vi "capture_dual_color_dual_view (SubVI).vi"(0 "SpimA path":path, 1 "Control values":T1, 2 "volume number":i32, 3 "filename prefix":string, 4 "Cam A handle in":u32, 5 "Capture on/off":bool, 6 "Cam A error in":errorcluster, 7 "Cam B error in":errorcluster, 8 "SpimB path":path, 10 "Cam B handle in":u32) -> (12 "Stage 0":u32, 14 "Stage 1":u32, 16 "Stage 2":u32, 18 "Stage 3":u32, 19 "Cam B Frame Count":i32, 20 "Camera A error out":errorcluster, 21 "DAC card stage A error":errorcluster, 22 "DAC card stage B error":errorcluster, 23 "interstage":u32, 24 "Camera A handle":u32, 25 "Camera B handle":u32, 26 "Cam A Frame Count":i32, 27 "Camera B error out":errorcluster)   [LabVIEW 2016]
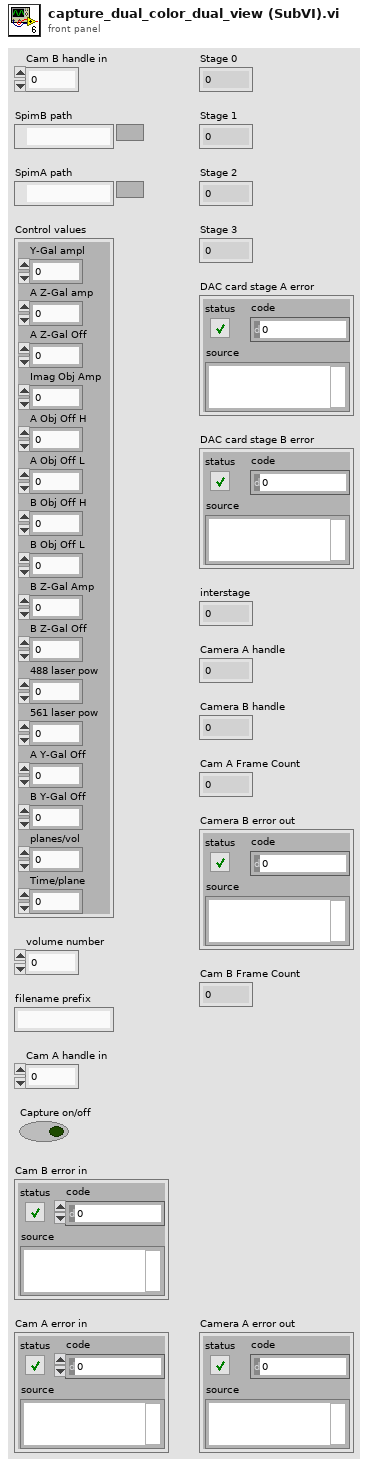
[diagram p1: front panel]
types:
  T1 = cluster{"Y-Gal ampl":dbl, "A Z-Gal amp":dbl, "A Z-Gal Off":dbl, "Imag Obj Amp":dbl, "A Obj Off H":dbl, "A Obj Off L":dbl, "B Obj Off H":dbl, "B Obj Off L":dbl, "B Z-Gal Amp":dbl, "B Z-Gal Off":dbl, "488 laser pow":dbl, "561 laser pow":dbl, "A Y-Gal Off":dbl, "B Y-Gal Off ":dbl, "planes/vol":dbl, "Time/plane":dbl}
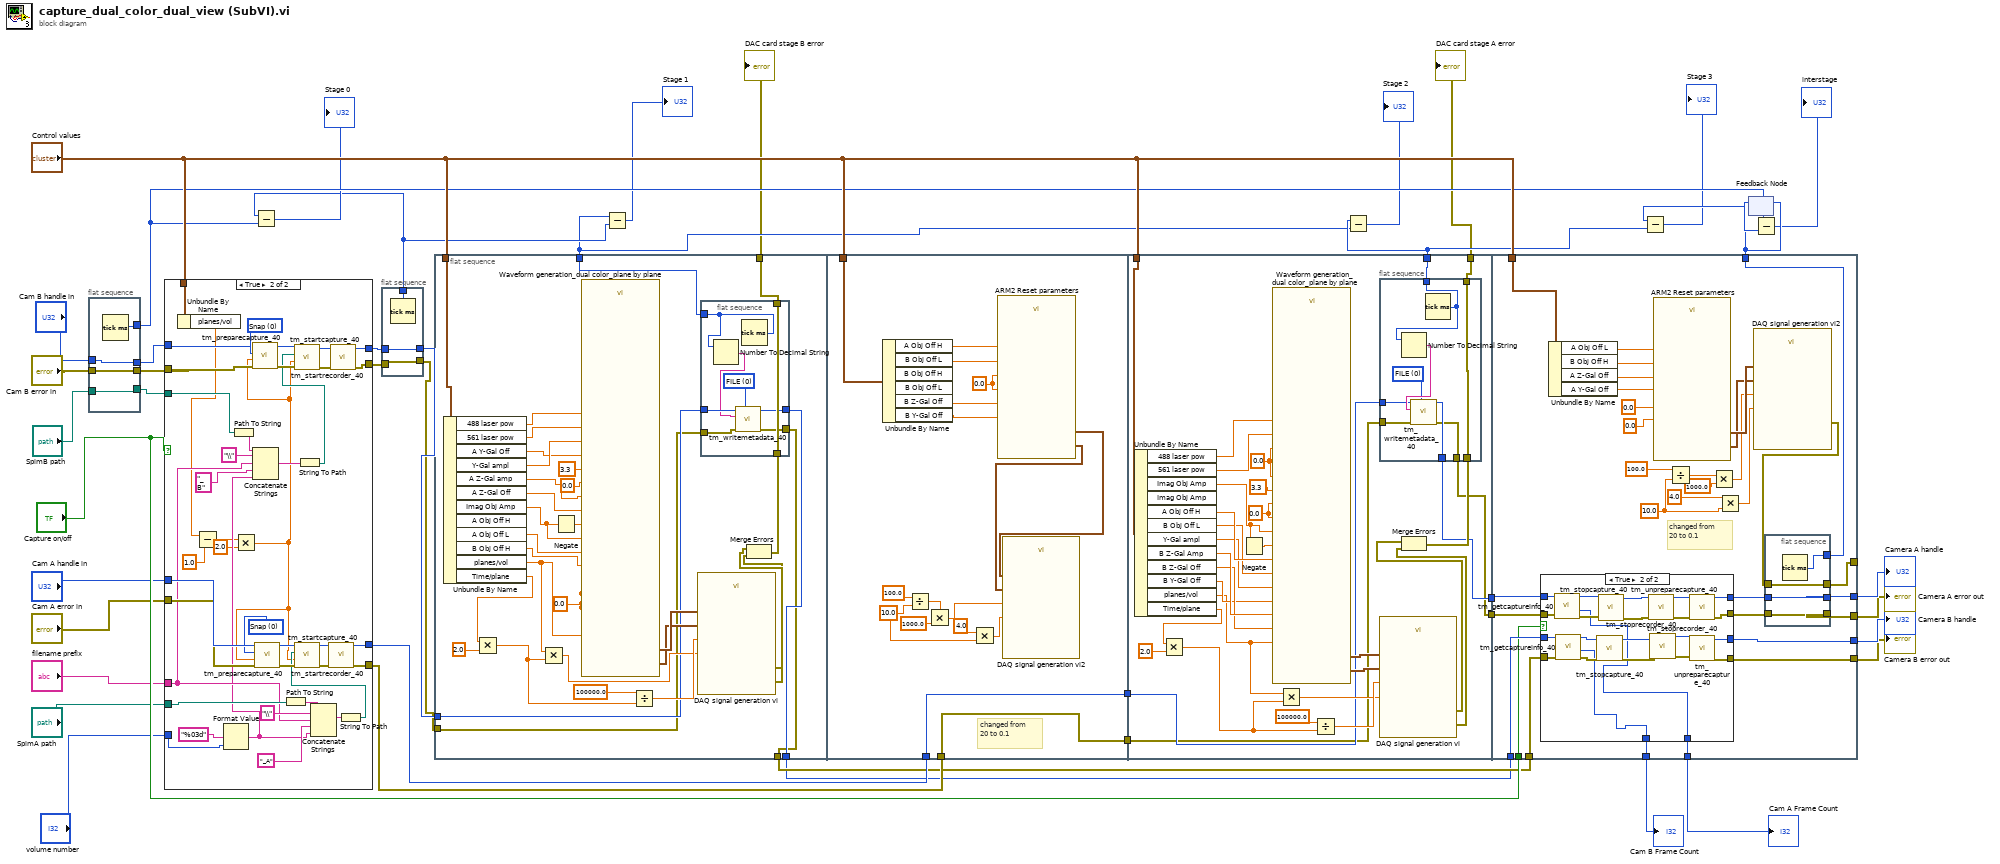
[diagram p0: block diagram]
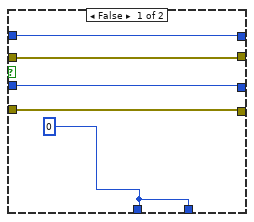
[diagram p3: hidden frame]
diagram:
  n1 = flat-sequence {
    tunnel: [w48] -> w19
    tunnel: "Cam B handle in" -> [w48]
    tunnel: [w47] -> w21
    tunnel: "Cam B error in" -> [w47]
    tunnel: [w46] -> w26
    tunnel: [w45] -> w35
    tunnel: "SpimB path" -> [w45]
    frame #0 {
      n2 = Tick Count (ms)() -> (millisecond timer value=w46:u32)
    }
  }
  n3 = case shown="True" "Capture on/off" {
    tunnel: "Cam A handle in" -> [w50 w86]
    tunnel: "Cam A error in" -> [w49 w85]
    tunnel: [w50 w77] -> w31
    tunnel: [w49 w75] -> w32
    tunnel: [w52 w82] -> w9
    tunnel: [w51 w81] -> w10
    tunnel: w19 -> [w52 w80]
    tunnel: w21 -> [w51 w79]
    tunnel: "SpimA path" -> [_ w68]
    tunnel: "volume number" -> [_ w67]
    tunnel: "filename prefix" -> [_ w60]
    tunnel: w35 -> [_ w58]
    tunnel: "Control values" -> [_ w57]
    frame False {
    }
    frame True {
      w83 = 0 items=["Snap", "Sequence"] ("Capture mode")
      w84 = 0 items=["Snap", "Sequence"] ("Capture mode")
      n4 = Unbundle By Name(w57) -> ("planes/vol"=w56:dbl)
      n5 = Subtract(x=w56, y=1.0) -> (x-y=w55:dbl)
      n6 = Format Value(format string="%03d", value (0)=w67) -> (output string=w59:string)  [unwired: 1 in]
      n7 = Path To String(path=w58) -> (string=w64:string)
      n8 = Multiply(x=w55, y=2.0) -> (x*y=w53:dbl)
      n9 = call <userlib>:"tm_preparecapture_40.vi"("error in (no error)"=w79, "Frames"=w53, "Capture mode"=w84, "Handle in"=w80) -> ("error out"=w90:errorcluster, "Handle out"=w89:u32)  [unwired: 4 in, 2 out]
      n10 = Concatenate Strings(w64, "\\", w60, "_B" ("string"), w59) -> (w63:string)
      n11 = call <userlib>:"tm_preparecapture_40.vi"("error in (no error)"=w85, "Frames"=w53, "Capture mode"=w83, "Handle in"=w86) -> ("error out"=w88:errorcluster, "Handle out"=w87:u32)  [unwired: 4 in, 2 out]
      n12 = Path To String(path=w68) -> (string=w72:string)
      n13 = String To Path(string=w63) -> (path=w61:path)
      n14 = call <userlib>:"tm_startrecorder_40.vi"("error in (no error)"=w90, "frames"=w53, "File"=w61, "Handle in"=w89) -> ("error out"=w92:errorcluster, "Handle out"=w91:u32)  [unwired: 6 in]
      n15 = Concatenate Strings(w72, "\\", w60, "_A" ("string"), w59) -> (w73:string)
      n16 = call <userlib>:"tm_startcapture_40.vi"("error in (no error)"=w92, "Handle in"=w91) -> ("error out"=w81:errorcluster, "Handle out"=w82:u32)  [unwired: 8 in]
      n17 = String To Path(string=w73) -> (path=w69:path)
      n18 = call <userlib>:"tm_startrecorder_40.vi"("error in (no error)"=w88, "frames"=w53, "File"=w69, "Handle in"=w87) -> ("error out"=w76:errorcluster, "Handle out"=w78:u32)  [unwired: 6 in]
      n19 = call <userlib>:"tm_startcapture_40.vi"("error in (no error)"=w76, "Handle in"=w78) -> ("error out"=w75:errorcluster, "Handle out"=w77:u32)  [unwired: 8 in]
    }
  }
  n20 = Subtract(x=w23, y=w26) -> (x-y=→"Stage 0":u32)
  n21 = flat-sequence {
    tunnel: [w95] -> w30
    tunnel: w9 -> [w95]
    tunnel: [w94] -> w28
    tunnel: w10 -> [w94]
    tunnel: [w93] -> w23
    frame #0 {
      n22 = Tick Count (ms)() -> (millisecond timer value=w93:u32)
    }
  }
  n23 = flat-sequence {
    tunnel: [w116] -> w3
    tunnel: [w112] -> w27
    tunnel: [w115] -> w13
    tunnel: w28 -> [w111]
    tunnel: [w110] -> w29
    tunnel: w30 -> [w113]
    tunnel: "Control values" -> [w109]
    tunnel: w31 -> [w142]
    tunnel: w32 -> [w141]
    tunnel: [w142] -> w44
    tunnel: [w141] -> w43
    tunnel: "Control values" -> [w140]
    tunnel: [w172] -> w42
    tunnel: [w171] -> w41
    tunnel: [w174] -> w8
    tunnel: [w173] -> w14
    tunnel: w44 -> [w170]
    tunnel: w43 -> [w169]
    tunnel: "Control values" -> [w167]
    tunnel: w42 -> [w223]
    tunnel: w41 -> [w222]
    tunnel: w29 -> [w224]
    tunnel: [w221] -> w4
    tunnel: [w220] -> w5
    tunnel: [w208] -> w6
    tunnel: [w206] -> w7
    tunnel: [w204] -> w17
    tunnel: [w203] -> _
    tunnel: w27 -> [w201]
    tunnel: "Control values" -> [w200]
    tunnel: "Capture on/off" -> [w195]
    tunnel: [w194] -> w39
    tunnel: [w193] -> w40
    frame #0 {
      w127 = 0.0 ("ARM2 Z-offset")
      n24 = Unbundle By Name(w109) -> ("488 laser pow"=w100:dbl, "561 laser pow"=w101:dbl, "A Y-Gal Off"=w102:dbl, "Y-Gal ampl"=w108:dbl, "A Z-Gal amp"=w107:dbl, "A Z-Gal Off"=w106:dbl, "Imag Obj Amp"=w105:dbl, "A Obj Off L"=w104:dbl, "B Obj Off H"=w103:dbl, "planes/vol"=w99:dbl, "Time/plane"=w97:dbl)  [unwired: 1 out]
      n25 = Multiply(x=w97, y=2.0) -> (x*y=w96:dbl)
      n26 = Multiply(x=w99, y=w96) -> (x*y=w121:dbl)
      n27 = Negate(x=w105) -> (-x=w114:dbl)
      n28 = call "Waveform generation_dual color_plane by plane.vi"("Number of Steps"=w99, "488 LASER Intensity"=w100, "SPIMA Obj Ampl"=w114, "SPIMB Z- galvo amplitude"=w127, "SPIMA Z-Galvo Offset"=w106, "SPIMA Z-Galvo Amplitude"=w107, "SPIMA Camera trigger"=0.0 ("ARM2 Camera trigger"), "SPIMA Obejective Offset"=w104, "SPIMB Obejective Offset"=w103, "SPIMA Y-Galvo Offset"=w102, "SPIMB Camera Trigger"=3.3 ("ARM1 Camera Trigger"), "561 Laser Amplitude"=w101, "SPIMB Objective Amplitude"=w105, "SPIMA Y-Galvo Amplitude"=w108, "SPIMB Z-offset"=w127, "SPIMB Y Offset"=w127, "SPIMB Y Amplitude"=w127) -> ("DAQ 2"=w125:waveform(dbl)[], "DAQ1"=w124:waveform(dbl)[])  [unwired: 9 in]
      n29 = Divide(x=100000.0, y=w96) -> (x/y=w122:dbl)
      n30 = call "DAQ signal generation vi.vi"("Time for each step"=w122, "Total time"=w121, "DAQ 1"=w124, "DAQ 2"=w125) -> ("error out"=w120:errorcluster, "error out 7"=w119:errorcluster)  [unwired: 6 in]
      n31 = flat-sequence {
        tunnel: w117 -> [w135]
        tunnel: [w135] -> w116
        tunnel: [w129] -> w115
        tunnel: w113 -> [w134]
        tunnel: [w133] -> w112
        tunnel: w111 -> [w132]
        tunnel: [w131] -> w110
        frame #0 {
          w130 = 0 items=["FILE"=0, "FRAME"=2] ("Type")
          n32 = Tick Count (ms)() -> (millisecond timer value=w129:u32)
          n33 = Number To Decimal String(number=w129) -> (decimal integer string=w128:string)  [unwired: 1 in]
          n34 = call <userlib>:"tm_writemetadata_40.vi"("Type"=w130, "error in (no error)"=w132, "Metadata"=w128, "Handle"=w134) -> ("error out"=w131:errorcluster, "Handle"=w133:u32)  [unwired: 6 in]
        }
      }
      n35 = Merge Errors(w120, w119) -> (w117:errorcluster)
    }
    frame #1 {
      w145 = 0.0 ("ARM1 Z-Galvo Offset")
      w149 = 10.0 ("y")
      # "changed from 20 to 0.1"
      n36 = Unbundle By Name(w140) -> ("A Obj Off H"=w139:dbl, "B Obj Off L"=w138:dbl, "B Z-Gal Off"=w137:dbl, "B Y-Gal Off"=w136:dbl)  [unwired: 2 out]
      n37 = Divide(x=100.0, y=w149) -> (x/y=w152:dbl)
      n38 = Multiply(x=w152, y=1000.0) -> (x*y=w147:dbl)
      n39 = Multiply(x=4.0, y=w149) -> (x*y=w146:dbl)
      n40 = call "ARM2 Reset parameters.vi"("ARM2 Y-Galvo Offset"=w136, "ARM2 Obejective Offset"=w138, "ARM2 Z-Galvo Offset"=w137, "ARM1 Z-Galvo Offset"=w145, "ARM1 Obejective Offset"=w139, "ARM1 Y-Galvo Offset"=w145) -> ("DAQ 2"=w144:waveform(dbl)[], "DAQ1"=w143:waveform(dbl)[])  [unwired: 8 in]
      n41 = call "DAQ signal generation vi2.vi"("Time for each step"=w147, "Total time"=w146, "DAQ1"=w143, "DAQ 2"=w144) -> ()  [unwired: 6 in, 2 out]
    }
    frame #2 {
      w168 = 0.0 ("SPIMB Camera Trigger")
      w176 = 0.0 ("ARM1 Y-Galvo Offset")
      n42 = Unbundle By Name(w167) -> ("488 laser pow"=w159:dbl, "561 laser pow"=w160:dbl, "Imag Obj Amp"=w157:dbl, "A Obj Off H"=w166:dbl, "B Obj Off L"=w165:dbl, "Y-Gal ampl"=w163:dbl, "B Z-Gal Amp"=w164:dbl, "B Z-Gal Off"=w162:dbl, "B Y-Gal Off"=w158:dbl, "planes/vol"=w156:dbl, "Time/plane"=w154:dbl)  [unwired: 1 out]
      n43 = Multiply(x=w154, y=2.0) -> (x*y=w153:dbl)
      n44 = Negate(x=w157) -> (-x=w161:dbl)
      n45 = call "Waveform generation_dual color_plane by plane.vi"("Number of Steps"=w156, "488 LASER Intensity"=w159, "SPIMA Obj Ampl"=w157, "SPIMB Z- galvo amplitude"=w164, "SPIMA Z-Galvo Offset"=w176, "SPIMA Z-Galvo Amplitude"=w176, "SPIMA Camera trigger"=3.3 ("ARM2 Camera trigger"), "SPIMA Obejective Offset"=w166, "SPIMB Obejective Offset"=w165, "SPIMA Y-Galvo Offset"=w168, "SPIMB Camera Trigger"=w168, "561 Laser Amplitude"=w160, "SPIMB Objective Amplitude"=w161, "SPIMA Y-Galvo Amplitude"=w168, "SPIMB Z-offset"=w162, "SPIMB Y Offset"=w158, "SPIMB Y Amplitude"=w163) -> ("DAQ 2"=w183:waveform(dbl)[], "DAQ1"=w182:waveform(dbl)[])  [unwired: 9 in]
      n46 = Multiply(x=w156, y=w153) -> (x*y=w179:dbl)
      n47 = Divide(x=100000.0, y=w153) -> (x/y=w180:dbl)
      n48 = flat-sequence {
        tunnel: [w192] -> w174
        tunnel: w175 -> [w192]
        tunnel: [w189] -> w173
        tunnel: [w191] -> w172
        tunnel: [w190] -> w171
        tunnel: w170 -> [w187]
        tunnel: w169 -> [w186]
        frame #0 {
          w185 = 0 items=["FILE"=0, "FRAME"=2] ("Type")
          n49 = Tick Count (ms)() -> (millisecond timer value=w189:u32)
          n50 = Number To Decimal String(number=w189) -> (decimal integer string=w188:string)  [unwired: 1 in]
          n51 = call <userlib>:"tm_writemetadata_40.vi"("Type"=w185, "error in (no error)"=w186, "Metadata"=w188, "Handle"=w187) -> ("error out"=w190:errorcluster, "Handle"=w191:u32)  [unwired: 6 in]
        }
      }
      n52 = call "DAQ signal generation vi.vi"("Time for each step"=w180, "Total time"=w179, "DAQ 1"=w182, "DAQ 2"=w183) -> ("error out"=w178:errorcluster, "error out 7"=w177:errorcluster)  [unwired: 6 in]
      n53 = Merge Errors(w178, w177) -> (w175:errorcluster)
    }
    frame #3 {
      w213 = 10.0 ("y")
      # "changed from 20 to 0.1"
      n54 = case shown="True" w195 {
        tunnel: w224 -> [w226 w239]
        tunnel: w223 -> [w229 w238]
        tunnel: w222 -> [w228 w237]
        tunnel: [w226 w236] -> w221
        tunnel: [w227 w235] -> w220
        tunnel: [w228 w234] -> w207
        tunnel: [w229 w233] -> w205
        tunnel: w201 -> [w227 w232]
        tunnel: [w225 w231] -> w194
        tunnel: [w225 w230] -> w193
        frame False {
          w225 = 0 ("Frame Count")
        }
        frame True {
          n55 = call <userlib>:"tm_getcaptureinfo_40.vi"("error in (no error)"=w237, "Handle in"=w238) -> ("error out"=w242:errorcluster, "Frame Count"=w230:i32, "Handle out"=w243:u32)  [unwired: 6 in, 1 out]
          n56 = call <userlib>:"tm_getcaptureinfo_40.vi"("error in (no error)"=w239, "Handle in"=w232) -> ("error out"=w240:errorcluster, "Frame Count"=w231:i32, "Handle out"=w241:u32)  [unwired: 6 in, 1 out]
          n57 = call <userlib>:"tm_stopcapture_40.vi"("error in (no error)"=w240, "Handle in"=w241) -> ("error out"=w246:errorcluster, "Handle out"=w247:u32)  [unwired: 8 in]
          n58 = call <userlib>:"tm_stopcapture_40.vi"("error in (no error)"=w242, "Handle in"=w243) -> ("error out"=w250:errorcluster, "Handle out"=w251:u32)  [unwired: 8 in]
          n59 = call <userlib>:"tm_stoprecorder_40.vi"("error in (no error)"=w250, "Handle in"=w251) -> ("error out"=w248:errorcluster, "Handle out"=w249:u32)  [unwired: 8 in]
          n60 = call <userlib>:"tm_stoprecorder_40.vi"("error in (no error)"=w246, "Handle in"=w247) -> ("error out"=w244:errorcluster, "Handle out"=w245:u32)  [unwired: 8 in]
          n61 = call <userlib>:"tm_unpreparecapture_40.vi"("error in (no error)"=w248, "Handle in"=w249) -> ("error out"=w234:errorcluster, "Handle out"=w233:u32)  [unwired: 8 in]
          n62 = call <userlib>:"tm_unpreparecapture_40.vi"("error in (no error)"=w244, "Handle in"=w245) -> ("error out"=w236:errorcluster, "Handle out"=w235:u32)  [unwired: 8 in]
        }
      }
      n63 = Unbundle By Name(w200) -> ("A Obj Off L"=w199:dbl, "B Obj Off H"=w198:dbl, "A Z-Gal Off"=w197:dbl, "A Y-Gal Off"=w196:dbl)
      n64 = call "ARM2 Reset parameters.vi"("ARM2 Y-Galvo Offset"=0.0, "ARM2 Obejective Offset"=w198, "ARM2 Z-Galvo Offset"=0.0, "ARM1 Z-Galvo Offset"=w197, "ARM1 Obejective Offset"=w199, "ARM1 Y-Galvo Offset"=w196) -> ("DAQ 2"=w219:waveform(dbl)[], "DAQ1"=w218:waveform(dbl)[])  [unwired: 8 in]
      n65 = Divide(x=100.0, y=w213) -> (x/y=w217:dbl)
      n66 = Multiply(x=w217, y=1000.0) -> (x*y=w211:dbl)
      n67 = Multiply(x=4.0, y=w213) -> (x*y=w212:dbl)
      n68 = call "DAQ signal generation vi2.vi"("Time for each step"=w211, "Total time"=w212, "DAQ1"=w218, "DAQ 2"=w219) -> ("error out"=w202:errorcluster)  [unwired: 6 in, 1 out]
      n69 = flat-sequence {
        tunnel: [w255] -> w208
        tunnel: w207 -> [w255]
        tunnel: [w254] -> w206
        tunnel: w205 -> [w254]
        tunnel: [w253] -> w204
        tunnel: [w252] -> w203
        tunnel: w202 -> [w252]
        frame #0 {
          n70 = Tick Count (ms)() -> (millisecond timer value=w253:u32)
        }
      }
    }
  }
  n71 = Subtract(x=w13, y=w23) -> (x-y=→"Stage 1":u32)
  n72 = Subtract(x=w14, y=w13) -> (x-y=→"Stage 2":u32)
  n73 = Subtract(x=w17, y=w14) -> (x-y=→"Stage 3":u32)
  n74 = feedback #1() -> (w18:u32)  [unwired: 1 in]
  n75 = feedback-in #1(w17) -> ()
  n76 = Subtract(x=w26, y=w18) -> (x-y=→"interstage":u32)
  "Cam A Frame Count" <- w40
  "Cam B Frame Count" <- w39
  "DAC card stage A error" <- w8
  "Camera A handle" <- w7
  "Camera A error out" <- w6
  "Camera B handle" <- w5
  "Camera B error out" <- w4
  "DAC card stage B error" <- w3
